vi "DAQmx Create Channel (AI-Acceleration-4 Wire DC Voltage).vi"(0 "task in":refnum<k21>, 1 "maximum value":dbl=5.0 format="%0.5f", 2 "minimum value":dbl=-5.0 format="%0.5f", 3 "input terminal configuration":i32(ring)=-1 items=["Default"=-1, "RSE"=10083, "NRSE"=10078, "Differential"=10106, "Pseudodifferential"=12529], 5 "physical channels":tag, 6 "use excitation for scaling":bool, 7 "name to assign":string, 8 "voltage excitation source":i32(ring)=10200 items=["Internal"=10200, "External"=10167, "None"=10230], 9 "units":i32(ring)=10186 items=["g"=10186, "m/s^2"=12470, "in/s^2"=12471, "From Custom Scale"=10065], 10 "voltage excitation value":dbl format="%.6f", 11 "error in":errorcluster, 12 "custom scale name":tag, 13 "sensitivity":dbl=1000.0, 14 "sensitivity units":i32(ring)=12509 items=["mVolts/g"=12509, "Volts/g"=12510]) -> (4 "task out":refnum<k21>, 15 "error out":errorcluster)   [LabVIEW 2013]
doc: "Creates channel(s) to measure acceleration. Use this instance for custom sensors that require excitation. You can use the excitation to scale the measurement."
uses:
  nilvaiu.dll
panel:
  # "input limits"
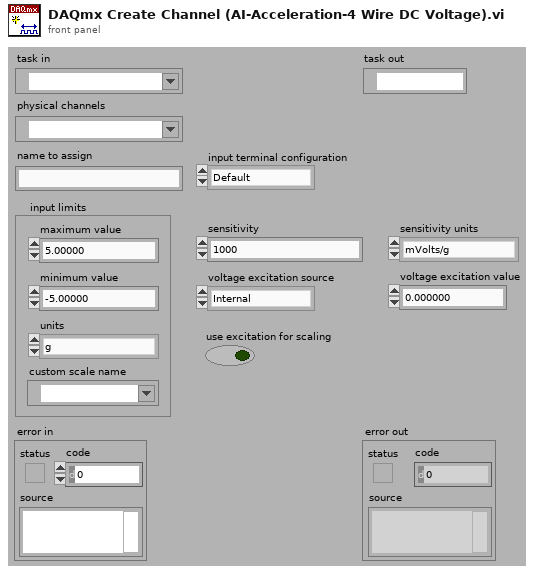
[diagram p1: front panel]
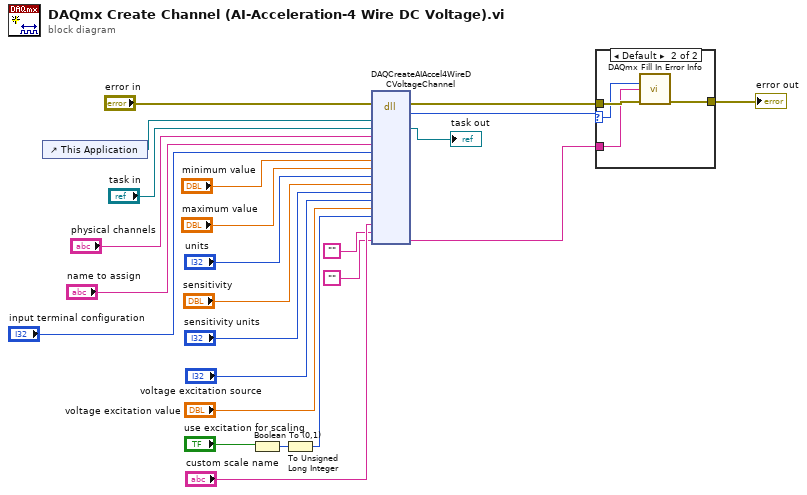
[diagram p0: block diagram]
diagram:
  n1 = control-ref of="This Application"() -> (w23:refnum<vi>)
  n2 = Boolean To (0,1)(Boolean="use excitation for scaling") -> (0, 1=w6:i16)
  n3 = To Unsigned Long Integer(number=w6) -> (unsigned 32bit integer=w4:u32)
  n4 = dll-call lib="nilvaiu.*" fn="DAQCreateAIAccel4WireDCVoltageChannel"(error in="error in", "lvAppReference"=w23, "taskID"="task in", "physical channel name"="physical channels", "virtual channel name"="name to assign", "input terminal configuration"="input terminal configuration", "minimum value"="minimum value", "maximum value"="maximum value", "units"="units", "sensitivity"="sensitivity", "sensitivity units"="sensitivity units", "voltage excitation source"="voltage excitation source", "voltage excitation value"="voltage excitation value", "use excitation for scaling"=w4, "customScale"="custom scale name", "channelNamesOut"="", "extendedErrorIndo"="") -> (error out=w13:errorcluster, "return type"=w11:i32, "taskID"=→"task out":refnum<k21>, "extendedErrorIndo"=w12:string)  [unwired: 16 in, 1 out]
  n5 = case shown="Default" w11 {
    selector: w11 -> [_ w27]
    tunnel: w13 -> [w25 w29]
    tunnel: [w25 w28] -> w14
    tunnel: w12 -> [_ w26]
    frame 0 {
    }
    frame Default {
      n6 = call "DAQmx Fill In Error Info.vi"("status code"=w27, "extended error info"=w26, "error in"=w29) -> ("error out"=w28:errorcluster)  [unwired: 1 in, 11 out]
    }
  }
  "error out" <- w14
